vi "Post-Dig.vi"(8 "Error In":errorcluster, 10 "Grave In":refnum<vi>, 11 "VI In":refnum<vi>) -> (0 "Error Out":errorcluster, 2 "Grave Out":refnum<vi>, 3 "VI Out":refnum<vi>)   [LabVIEW 2018, in "Tests.lvlib" / "Toolkit.lvlib" / "Integration.lvlib"]
uses:
  Integration.lvlib
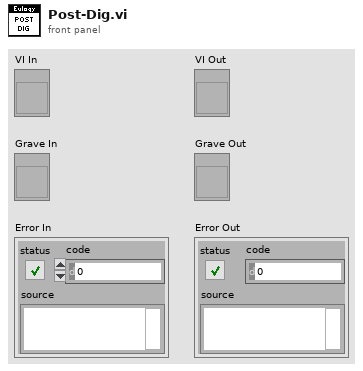
[diagram p1: front panel]
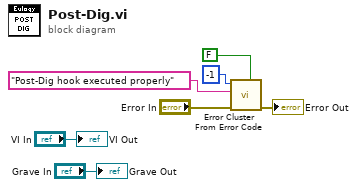
[diagram p0: block diagram]
diagram:
  n1 = call <vilib>:"Error Cluster From Error Code.vi"("is warning? (False)"=FALSE, "error in (no error)"="Error In", "error message (\"\")"="Post-Dig hook executed properly" ("error message (\"\")"), "error code (0)"=-1) -> ("error out"=→"Error Out":errorcluster)  [unwired: 5 in]
  "VI Out" <- "VI In"
  "Grave Out" <- "Grave In"
